vi "Update_TrainingExamples.vi"(8 "error in (no error)":errorcluster) -> (0 "error out":errorcluster, 2 "training number":string[][](array[string]), 3 "package":string[](array[string]))   [LabVIEW 2019]
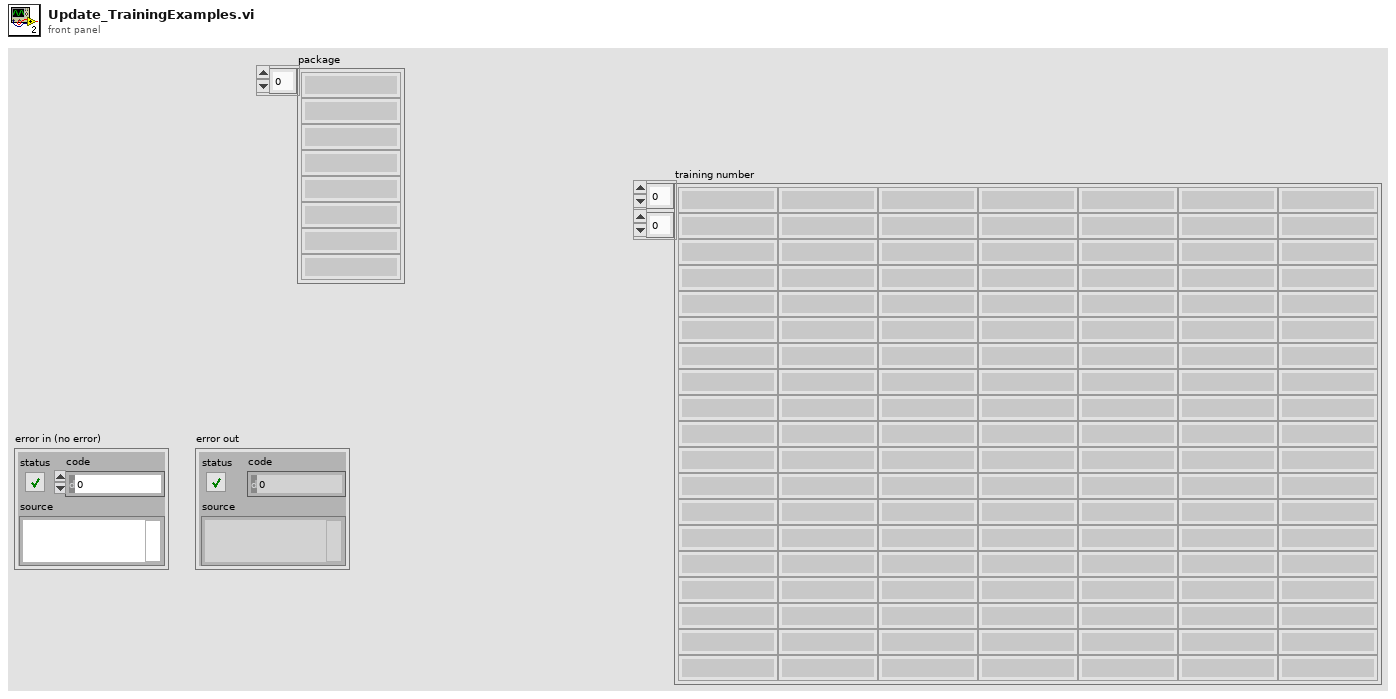
[diagram p1: front panel]
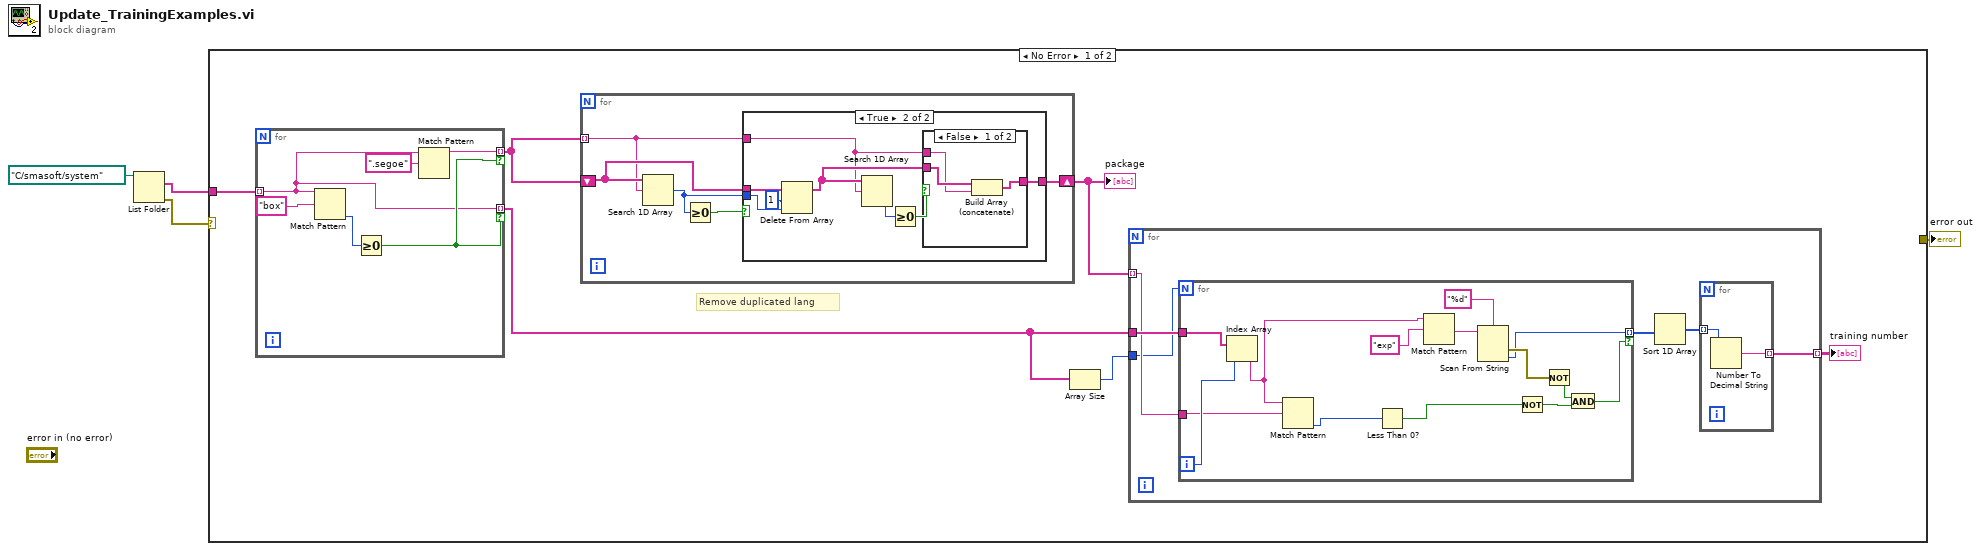
[diagram p0: block diagram]
diagram:
  n1 = List Folder(path=path "C:/smasoft/system") -> (filenames=w1:string[], error out=w3:errorcluster)  [unwired: 3 in, 2 out]
  n2 = case shown="No Error" w3 {
    selector: w3 -> [_ w57]
    tunnel: w1 -> [w10 _]
    tunnel: [_ w57] -> w2
    frame No Error {
      # "Remove duplicated lang"
      n3 = for {
        tunnel: w10 -> [w51] mode=indexing
        tunnel: [w51] -> w8 mode=indexing if=w52
        tunnel: [w53] -> w9 mode=indexing if=w52
        n4 = Match Pattern(string=w51, regular expression="box") -> (offset past match=w55:i32)  [unwired: 1 in, 3 out]
        n5 = Greater Or Equal To 0?(x=w55) -> (x >= 0?=w52:bool)
        n6 = Match Pattern(string=w51, regular expression=".segoe") -> (before substring=w53:string)  [unwired: 1 in, 3 out]
      }
      n7 = for {
        tunnel: w9 -> [w33] mode=indexing
        shift-right: [w35] -> w6
        shift-left: w9 -> [w37]
        n8 = Search 1D Array(1D array=w37, element=w33) -> (index of element=w36:i32)  [unwired: 1 in]
        n9 = Greater Or Equal To 0?(x=w36) -> (x >= 0?=w34:bool)
        n10 = case shown="True" w34 {
          tunnel: w37 -> [w38 w46]
          tunnel: w36 -> [_ w45]
          tunnel: [w38 w41] -> w35
          tunnel: w33 -> [_ w39]
          frame False {
          }
          frame True {
            n11 = Delete From Array(array=w46, length=1, index=w45) -> (array with subset deleted=w40:string[])  [unwired: 1 out]
            n12 = Search 1D Array(1D array=w40, element=w39) -> (index of element=w43:i32)  [unwired: 1 in]
            n13 = Greater Or Equal To 0?(x=w43) -> (x >= 0?=w42:bool)
            n14 = case shown="False" w42 {
              tunnel: [w47 w50] -> w41
              tunnel: w40 -> [w49 w50]
              tunnel: w39 -> [w48 _]
              frame False {
                n15 = Build Array (concatenate)(w49, w48) -> (w47:string[])
              }
              frame True {
              }
            }
          }
        }
      }
      "package" <- w6
      n16 = Array Size(array=w8) -> (size(s)=w7:i32)
      n17 = for {
        tunnel: w6 -> [w15] mode=indexing
        tunnel: w8 -> [w16]
        tunnel: w7 -> [w14]
        tunnel: [w11] -> w5 mode=indexing
        n18 = for {
          N: w14 -> [_]
          tunnel: w16 -> [w27]
          tunnel: w15 -> [w25]
          tunnel: [w19] -> w13 mode=indexing if=w22
          i -> [w26]
          n19 = Index Array(array=w27, index=w26) -> (element=w23:string)
          n20 = Match Pattern(string=w23, regular expression=w25) -> (offset past match=w24:i32)  [unwired: 1 in, 3 out]
          n21 = Less Than 0?(x=w24) -> (x < 0?=w29:bool)
          n22 = Match Pattern(string=w23, regular expression="exp") -> (after substring=w31:string)  [unwired: 1 in, 3 out]
          n23 = Scan From String(format string="%d", input string=w31) -> (error out=w21:errorcluster, output 1=w19:i32)  [unwired: 3 in, 2 out]
          n24 = Not(x=w29) -> (.not. x?=w28:bool)
          n25 = Not(x=w21) -> (.not. x?=w20:bool)
          n26 = And(x=w20, y=w28) -> (x .and. y?=w22:bool)
        }
        n27 = Sort 1D Array(array=w13) -> (sorted array=w12:i32[])
        n28 = for {
          tunnel: w12 -> [w18] mode=indexing
          tunnel: [w17] -> w11 mode=indexing
          n29 = Number To Decimal String(number=w18) -> (decimal integer string=w17:string)  [unwired: 1 in]
        }
      }
      "training number" <- w5
    }
    frame Error {
    }
  }
  "error out" <- w2
